vi "GetVariableFiles.vi"(10 "Ftp":refnum<k24>, 11 "error in":errorcluster) -> (3 "error out":errorcluster)   [LabVIEW 2011, in "UnderAutomation.Fanuc.lvlib"]
uses:
  UnderAutomation.Fanuc.lvlib
  C:/Users/fg/Documents/Fanuc.vi/LabVIEW_2024/UnderAutomation.Fanuc/lib/UnderAutomation.Fanuc.dll
  LabVIEW_2024/UnderAutomation.Fanuc/lib/UnderAutomation.Fanuc.dll
panel:
  out "VariableFiles":string[](array[string])
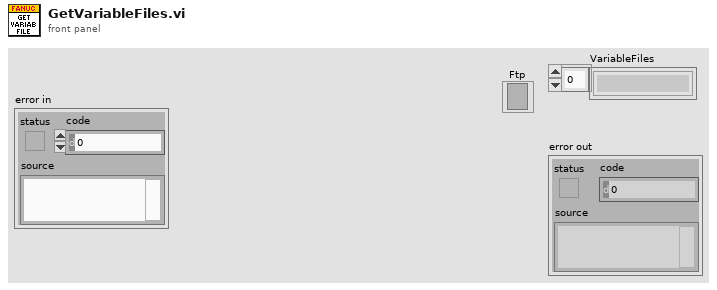
[diagram p1: front panel]
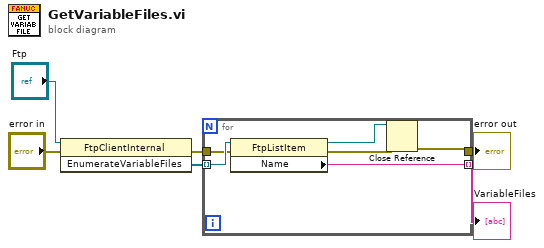
[diagram p0: block diagram]
diagram:
  n1 = invoke class="FtpClientInternal" method="EnumerateVariableFiles"(reference="Ftp", error in="error in") -> (error out=w3:errorcluster, "EnumerateVariableFiles"=w5:refnum<k24>[])  [unwired: 1 in, 1 out]
  n2 = for {
    tunnel: w5 -> [w12] mode=indexing
    tunnel: [w11] -> w4 mode=indexing
    tunnel: w3 -> [w10]
    tunnel: [w8] -> w2
    n3 = property class="FtpListItem"(reference=w12, error in=w10) -> (reference out=w7:refnum<k24>, error out=w9:errorcluster, "Name"=w11:string)
    n4 = Close Reference(reference=w7, error in (no error)=w9) -> (error out=w8:errorcluster)
  }
  "error out" <- w2
  "VariableFiles" <- w4
